vi "UE9 Multiple IO Example.vi"() -> ()   [LabVIEW 2021]
panel:
  out "Read Values":T1 {"AIN3" format="%.6f"; "AIN2" format="%.6f"; "AIN1" format="%.6f"; "AIN0" format="%.6f"}
  in  "Write Values":T2 {"DAC1" format="%.4f"; "DAC0" format="%.4f"}
  out "Error Message":string
  in  "error in":errorcluster
  out "error out":errorcluster
  # "Outputs DAC0-DAC1 and FIO2-FIO3.  Aquires AIN0-AIN3 and FIO0-FIO1.  Uses USB on the first found UE9."
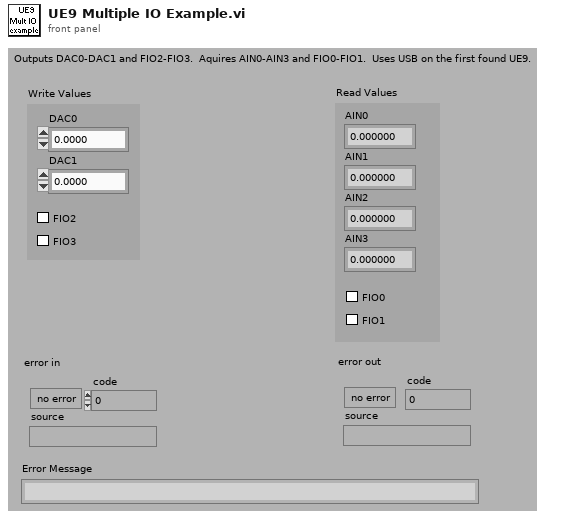
[diagram p1: front panel]
types:
  T1 = cluster{"AIN0":dbl, "AIN1":dbl, "AIN2":dbl, "AIN3":dbl, "FIO0":bool, "FIO1":bool}
  T2 = cluster{"DAC0":dbl, "DAC1":dbl, "FIO2":bool, "FIO3":bool}
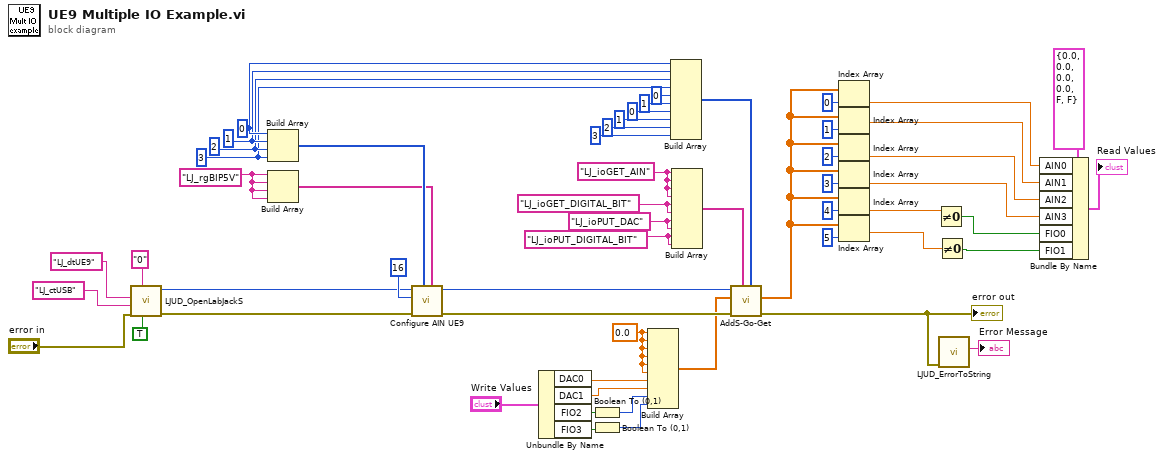
[diagram p0: block diagram]
diagram:
  w35 = 0.0 ("Input Element")
  w48 = "LJ_ioPUT_DIGITAL_BIT" ("IOType")
  w49 = "LJ_ioPUT_DAC" ("IOType")
  w51 = "LJ_ioGET_AIN" ("IOType")
  w44 = 3 ("SettlingFactor")
  w45 = 2 ("SettlingFactor")
  w46 = 1 ("SettlingFactor")
  w47 = 0 ("SettlingFactor")
  w20 = "LJ_rgBIP5V" ("AIN Range")
  w50 = "LJ_ioGET_DIGITAL_BIT" ("IOType")
  n1 = call "LJUD_OpenLabJackS.vi"("FirstFound"=TRUE, "Address"="0", "error in"="error in", "ConnectionType"="LJ_ctUSB", "DeviceType"="LJ_dtUE9") -> ("error out"=w22:errorcluster, "Handle"=w18:i32)  [unwired: 4 in, 1 out]
  n2 = Build Array(w47, w46, w45, w44) -> (w21:i32[])
  n3 = Build Array(w20, w20, w20, w20) -> (w19:string[])
  n4 = call "Configure AIN UE9.vi"("Ranges"=w19, "Channels"=w21, "error in"=w22, "Resolution"=16, "Handle In"=w18) -> ("error out"=w54:errorcluster, "Handle Out"=w55:i32)  [unwired: 5 in]
  n5 = Unbundle By Name("Write Values") -> ("DAC0"=w30:dbl, "DAC1"=w29:dbl, "FIO2"=w28:bool, "FIO3"=w27:bool)
  n6 = Boolean To (0,1)(Boolean=w28) -> (0, 1=w34:i16)
  n7 = Boolean To (0,1)(Boolean=w27) -> (0, 1=w33:i16)
  n8 = Build Array(w35, w35, w35, w35, w35, w35, w30, w29, w34, w33) -> (w32:dbl[])
  n9 = Build Array(w47, w46, w45, w44, 0 ("Input Element"), 1 ("Input Element"), 0 ("Input Element"), 1 ("Input Element"), 2 ("Input Element"), 3 ("Input Element")) -> (w36:i32[])
  n10 = Build Array(w51, w51, w51, w51, w50, w50, w49, w49, w48, w48) -> (w37:string[])
  n11 = call "AddS-Go-Get.vi"("Channels"=w36, "IOTypes"=w37, "error in"=w54, "Values Write"=w32, "Handle In"=w55) -> ("error out"=w53:errorcluster, "Values Read"=w8:dbl[])  [unwired: 4 in, 1 out]
  "error out" <- w53
  n12 = Index Array(array=w8, index=0 ("Index")) -> (element=w6:dbl)
  n13 = Index Array(array=w8, index=1 ("Index")) -> (element=w5:dbl)
  n14 = Index Array(array=w8, index=2 ("Index")) -> (element=w4:dbl)
  n15 = Index Array(array=w8, index=3 ("Index")) -> (element=w3:dbl)
  n16 = Index Array(array=w8, index=4 ("Index")) -> (element=w2:dbl)
  n17 = Index Array(array=w8, index=5 ("Index")) -> (element=w1:dbl)
  n18 = Not Equal To 0?(x=w2) -> (x != 0?=w23:bool)
  n19 = Not Equal To 0?(x=w1) -> (x != 0?=w24:bool)
  n20 = call "LJUD_ErrorToString.vi"("error in"=w53) -> ("String"=→"Error Message":string)  [unwired: 10 in]
  n21 = Bundle By Name(cluster=T1 {"AIN0"=0.0, "AIN1"=0.0, "AIN2"=0.0, "AIN3"=0.0, "FIO0"=FALSE, "FIO1"=FALSE} ("Read Values"), "AIN0"=w6, "AIN1"=w5, "AIN2"=w4, "AIN3"=w3, "FIO0"=w23, "FIO1"=w24) -> (→"Read Values":T1)
